vi "dl950_wave_20240509.vi"() -> ()   [LabVIEW 2019]
uses:
  950b817e-b14a-4b5d-8110-72b26e05e848.vi
  <instrlib>/Yokogawa DL950 Series/Public/Configure/Configure Module (4-CH Voltage).vi
  <instrlib>/Yokogawa DL950 Series/Public/Data/Read Waveform (Multiple).vi
  <instrlib>/Yokogawa DL950 Series/Yokogawa DL950 Series.lvlib
panel:
  out "Discharge":bool
  out "Power Relay":bool=TRUE
  out "Compute":bool
  out "DL950 Trigger":bool
  out "Power":bool=TRUE
  out "Ch 4":bool
  out "Ch 3":bool=TRUE
  out "Ch 2":bool
  out "Ch 1":bool
  in  "Channel Enale(1: CH1)":u16[](array[ring])=[1, 1] items=["", "CH1", "CH2", "CH3", "CH4", "CH5", "CH6", "CH7", "CH8", "CH9", "CH10", "CH11", "CH12", "CH13", "CH14", "CH15", "CH16", "RMATH1", "RMATH2", "RMATH3", "RMATH4", "RMATH5", "RMATH6", "RMATH7", "RMATH8", "RMATH9", "RMATH10", "RMATH11", "RMATH12", "RMATH13", "RMATH14", "RMATH15", "RMATH16"]
  in  "channel":i32[](array[ring])=[1, 2] items=["", "CH1_1", "CH1_2", "CH2_1", "CH2_2", "CH3_1", "CH3_2", "CH4_1", "CH4_2", "CH5_1", "CH5_2", "CH6_1", "CH6_2", "CH7_1", "CH7_2", "CH8_1", "CH8_2", "CH9_1", "CH9_2", "CH10_1", "CH10_2", "CH11_1", "CH11_2", "CH12_1", "CH12_2", "CH13_1", "CH13_2", "CH14_1", "CH14_2", "CH15_1", "CH15_2", "CH16_1", "CH16_2"]
  in  "trig source":i32[](array[ring])=[1, 1] items=["", "CH1", "CH2", "CH3", "CH4", "CH5", "CH6", "CH7", "CH8", "CH9", "CH10", "CH11", "CH12", "CH13", "CH14", "CH15", "CH16", "RMATH1", "RMATH2", "RMATH3", "RMATH4", "RMATH5", "RMATH6", "RMATH7", "RMATH8", "RMATH9", "RMATH10", "RMATH11", "RMATH12", "RMATH13", "RMATH14", "RMATH15", "RMATH16"]
  in  "sub channel":u16[](array[ring])=[1, 2] items=["None", "SCH1", "SCH2", "SCH3", "SCH4", "SCH5", "SCH6", "SCH7", "SCH8", "SCH9", "SCH10", "SCH11", "SCH12", "SCH13", "SCH14", "SCH15", "SCH16", "SCH17", "SCH18", "SCH19", "SCH20", "SCH21", "SCH22", "SCH23", "SCH24", "SCH25", "SCH26", "SCH27", "SCH28", "SCH29", "SCH30", "SCH31", "SCH32", "SCH33", "SCH34", "SCH35", "SCH36", "SCH37", "SCH38", "SCH39", "SCH40", "SCH41", "SCH42", "SCH43", "SCH44", "SCH45", "SCH46", "SCH47", "SCH48", "SCH49", "SCH50", "SCH51", "SCH52", "SCH53", "SCH54", "SCH55", "SCH56", "SCH57", "SCH58", "SCH59", "SCH60", "SCH61", "SCH62", "SCH63", "SCH64"]
  in  "Vertical Division (20: 50V)":i32(ring)=11 items=["0.1m", "0.2m", "0.5m", "1m", "2m", "5m", "10m", "20m", "50m", "100m", "200m", "500m", "1", "2", "4", "5", "8", "10", "20", "40", "50", "80", "100", "200", "400", "500", "800", "1k", "2k", "4k", "5k", "8k", "10k", "20k", "25k", "50k", "100k", "250k", "500k", "1000k"]
  in  "Hysteresis (1: Middle)":i32(ring)=1 items=["Low", "Middle", "High"]
  in  "Trigger Level (0)":dbl=0.4 format="%.3p"
  in  "Trigger Slope (0: Rising)":i32(ring) items=["Rising", "Falling", "Both"]
  in  "Trigger Mode (1: Auto)":i32(ring)=2 items=["Normal", "Auto", "Auto Level", "Single", "Single(N)", "On Start", "No Set"]
  in  "Time Division (12: 1ms)":i32(ring)=18 items=["100ns", "200ns", "500ns", "1us", "2us", "5us", "10us", "20us", "50us", "100us", "200us", "500us", "1ms", "2ms", "5ms", "10ms", "20ms", "50ms", "100ms", "200ms", "500ms", "1s", "2s", "3s", "4s", "5s", "6s", "10s", "20s", "30s", "1min", "2min", "3min", "4min", "5min", "6min", "10min", "12min", "30min", "1hour", "2hour", "3hour", "4hour", "5hour", "6hour", "8hour", "10hour", "12hour", "1day", "2day", "3day", "4day", "5day"]
  in  "Acquisition Mode (0: Normal)":i32(ring) items=["Normal", "Average", "Envelope"]
  in  "Record Length (0: 10k)":i32(ring) items=["10k", "25k", "50k", "100k", "250k", "500k", "1M", "2.5M", "5M", "10M", "25M", "50M", "100M", "250M", "500M", "1G", "2G", "4G", "5G", "10G", "20G", "50G"]
  in  "Sub Channel (0: None) 2":u16[](array[ring])=[1, 2] caption="Sub Channel (0: None)" items=["None", "SCH1", "SCH2", "SCH3", "SCH4", "SCH5", "SCH6", "SCH7", "SCH8", "SCH9", "SCH10", "SCH11", "SCH12", "SCH13", "SCH14", "SCH15", "SCH16", "SCH17", "SCH18", "SCH19", "SCH20", "SCH21", "SCH22", "SCH23", "SCH24", "SCH25", "SCH26", "SCH27", "SCH28", "SCH29", "SCH30", "SCH31", "SCH32", "SCH33", "SCH34", "SCH35", "SCH36", "SCH37", "SCH38", "SCH39", "SCH40", "SCH41", "SCH42", "SCH43", "SCH44", "SCH45", "SCH46", "SCH47", "SCH48", "SCH49", "SCH50", "SCH51", "SCH52", "SCH53", "SCH54", "SCH55", "SCH56", "SCH57", "SCH58", "SCH59", "SCH60", "SCH61", "SCH62", "SCH63", "SCH64"]
  in  "Source (1: CH1) 2":u16[](array[ring])=[1, 1] caption="Source (1: CH1)" items=["None", "CH1", "CH2", "CH3", "CH4", "CH5", "CH6", "CH7", "CH8", "CH9", "CH10", "CH11", "CH12", "CH13", "CH14", "CH15", "CH16", "MATH1", "MATH2", "MATH3", "MATH4", "MATH5", "MATH6", "MATH7", "MATH8", "EVENT"]
  in  "Probe Attenuation (3: 10:1)":i32(ring)=3 caption="Probe (10: 1)" items=["1:1", "2:1", "5:1", "10:1", "20:1", "50:1", "100:1", "200:1", "500:1", "1000:1", "2000:1", "5000:1", "10k:1", "20k:1", "50k:1", "0.1A:1V", "0.2A:1V", "0.5A:1V", "1A:1V", "2A:1V", "5A:1V", "10A:1V", "20A:1V", "50A:1V", "100A:1V", "200A:1V", "250A:1V", "400A:1V", "500A:1V", "1kA:1V", "2kA:1V", "5kA:1V", "10kA:1V", "20kA:1V", "50kA:1V", "NoSet"]
  in  "Vertical Coupling (1: DC)":i32(ring)=1 items=["AC", "DC", "Ground", "AC-RMS", "DC-RMS"]
  out "x-y":u32=4302
  in  "Enable Calibration (F: No)":bool
  in  "Enable Auto Setup (T: Yes)":bool
  in  "VISA resource name":refnum<visa-resource-name>="TCPIP0::192.168.0.100::inst0::INSTR"
  out "Waveform Graph":waveform(dbl)[](graph)=[{"t0"=timestamp(0 s since 1904-01-01), "dt"=0.0001, "Y"=array[10001 elements]}, {"t0"=timestamp(0 s since 1904-01-01), "dt"=0.0001, "Y"=array[10001 elements]}]
  in  "stop":bool
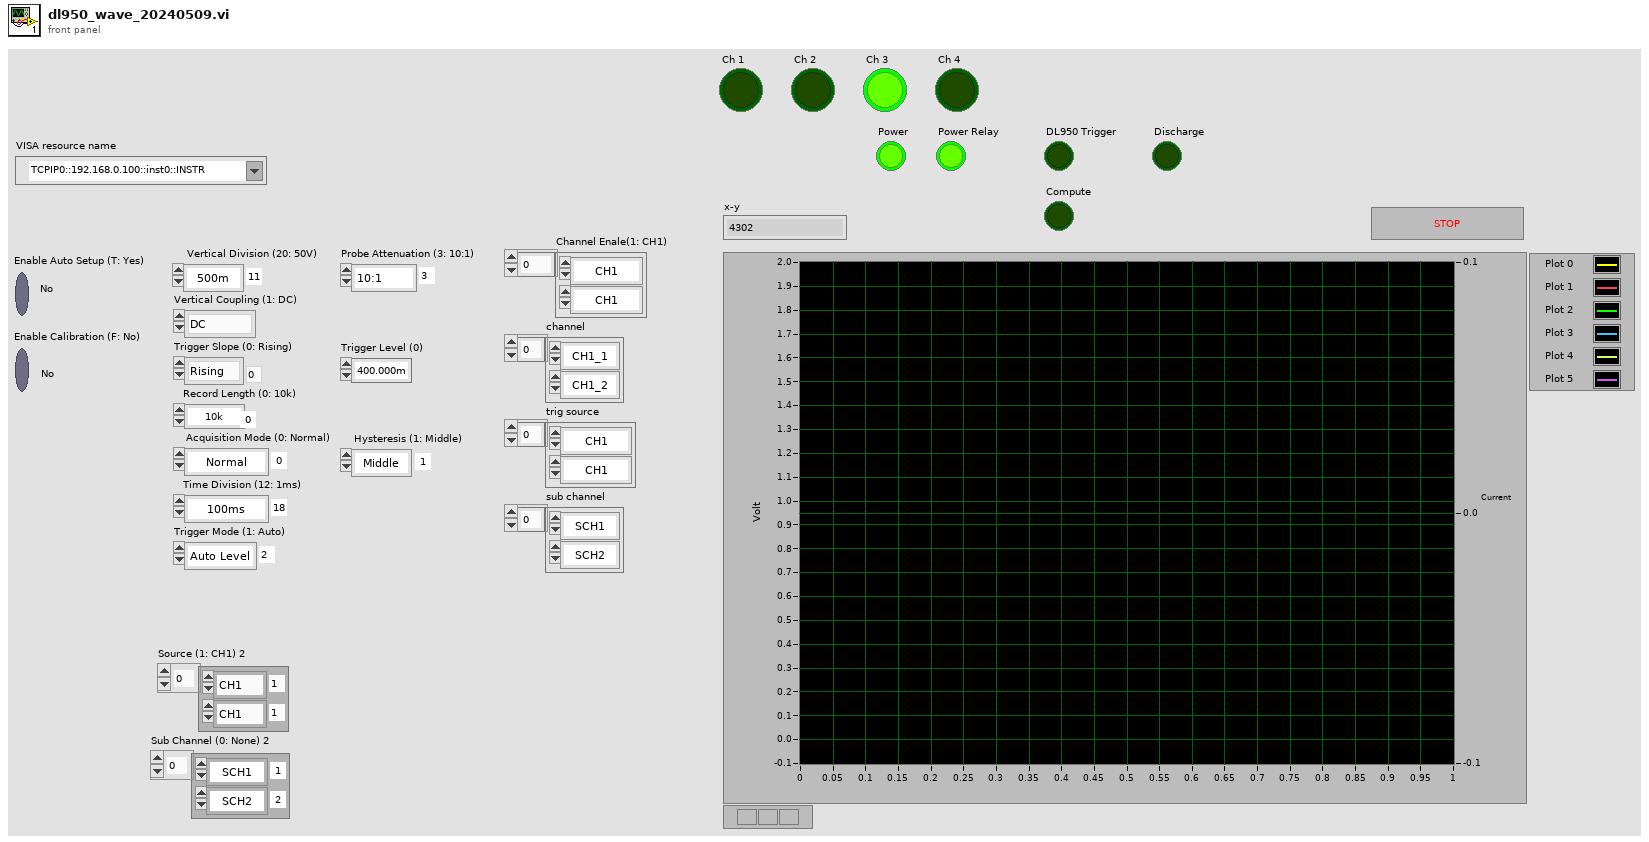
[diagram p1: front panel]
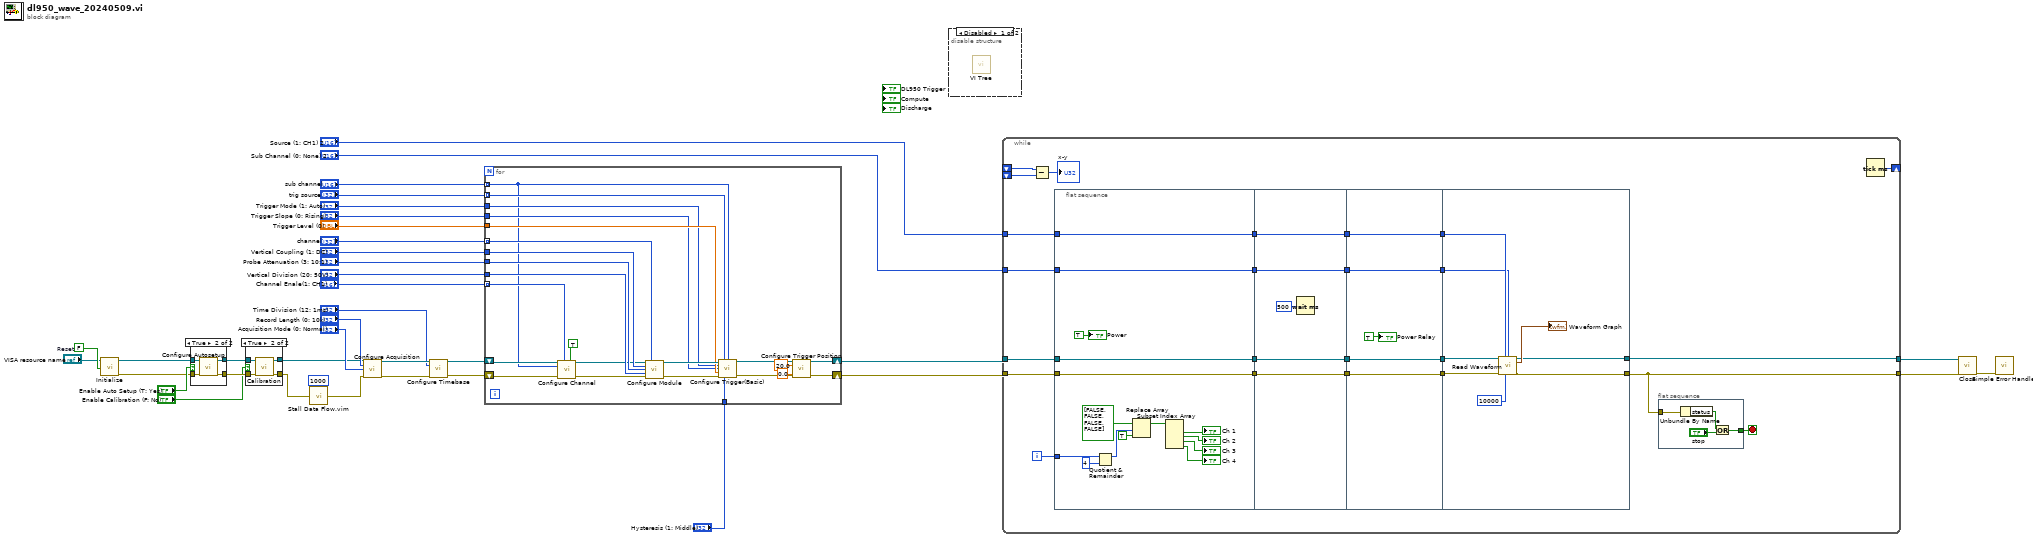
[diagram p0: block diagram]
diagram:
  w37 = FALSE  # Reset
  n1 = call <instrlib>:"Initialize.vi"("Reset (True)"=w37, "VISA resource name"="VISA resource name") -> ("error out"=w4:errorcluster, "VISA resource name out"=w5:refnum<visa-resource-name>)  [unwired: 8 in]
  n2 = case shown="True" "Enable Auto Setup (T: Yes)" {
    tunnel: w5 -> [w39 w43]
    tunnel: [w39 w42] -> w33
    tunnel: w4 -> [w38 w41]
    tunnel: [w38 w40] -> w32
    frame False {
    }
    frame True {
      n3 = call <instrlib>:"Configure Autosetup.vi"("VISA resource name"=w43, "error in (no error)"=w41) -> ("VISA resource name out"=w42:refnum<visa-resource-name>, "error out"=w40:errorcluster)  [unwired: 12 in]
    }
  }
  n4 = case shown="True" "Enable Calibration (F: No)" {
    tunnel: w33 -> [w45 w49]
    tunnel: [w45 w48] -> w3
    tunnel: w32 -> [w44 w47]
    tunnel: [w44 w46] -> w2
    frame False {
    }
    frame True {
      n5 = call <instrlib>:"Calibration.vi"("error in (no error)"=w47, "VISA resource name"=w49) -> ("error out"=w46:errorcluster, "VISA resource name out"=w48:refnum<visa-resource-name>)  [unwired: 8 in]
    }
  }
  n6 = call "Stall Data Flow.vim"("value in"=w2, "milliseconds to wait"=u32 1000) -> ("value out"=w1:errorcluster)  [unwired: 1 out]
  n7 = call <instrlib>:"Configure Acquisition.vi"("VISA resource name"=w3, "Record Length (0: 10k)"="Record Length (0: 10k)", "Acquisition Mode (0: Normal)"="Acquisition Mode (0: Normal)", "error in (no error)"=w1) -> ("VISA resource name out"=w24:refnum<visa-resource-name>, "error out"=w23:errorcluster)  [unwired: 10 in]
  n8 = call <instrlib>:"Configure Timebase.vi"("VISA resource name"=w24, "Time Division (12: 1ms)"="Time Division (12: 1ms)", "error in (no error)"=w23) -> ("VISA resource name out"=w22:refnum<visa-resource-name>, "error out"=w21:errorcluster)  [unwired: 11 in]
  n9 = for {
    tunnel: "channel" -> [w60] mode=indexing
    tunnel: "trig source" -> [w73] mode=indexing
    tunnel: "sub channel" -> [w56] mode=indexing
    tunnel: "Hysteresis (1: Middle)" -> [w72]
    shift-right: [w54] -> w7
    shift-left: w22 -> [w63]
    shift-right: [w52] -> w6
    shift-left: w21 -> [w61]
    tunnel: "Trigger Level (0)" -> [w69]
    tunnel: "Trigger Slope (0: Rising)" -> [w68]
    tunnel: "Trigger Mode (1: Auto)" -> [w67]
    tunnel: "Vertical Division (20: 50V)" -> [w66]
    tunnel: "Probe Attenuation (3: 10:1)" -> [w65]
    tunnel: "Vertical Coupling (1: DC)" -> [w64]
    tunnel: "Channel Enale(1: CH1)" -> [w58] mode=indexing
    n10 = call <instrlib>:"Configure Channel.vi"("VISA resource name"=w63, "Channel (1: CH1)"=w58, "Enable Channel (True)"=TRUE, "sub Channel (1: CH1)"=w56, "error in (no error)"=w61) -> ("VISA resource name out"=w62:refnum<visa-resource-name>, "error out"=w59:errorcluster)  [unwired: 9 in]
    n11 = call-poly <instrlib>:"Configure Module.vi"("VISA resource name"=w62, "Channel (1: CH1_1)"=w60, "Vertical Coupling (1: DC)"=w64, "Probe Attenuation (3: 10:1)"=w65, "Vertical Division (20: 50V)"=w66, "error in (no error)"=w59) -> ("VISA resource name out"=w71:refnum<visa-resource-name>, "error out"=w70:errorcluster)  [unwired: 8 in]
    n12 = call <instrlib>:"Configure Trigger(Basic).vi"("VISA resource name"=w71, "Trigger Source (1: CH1)"=w73, "Sub Channel (0: None)"=w56, "Trigger Mode (1: Auto)"=w67, "Trigger Slope (0: Rising)"=w68, "Trigger Level (0)"=w69, "error in (no error)"=w70, "Hysteresis (1: Middle)"=w72) -> ("VISA resource name out"=w55:refnum<visa-resource-name>, "error out"=w53:errorcluster)  [unwired: 6 in]
    n13 = call <instrlib>:"Configure Trigger Position.vi"("VISA resource name"=w55, "Trigger Position (50%)"=20.0, "Trigger Delay (0.0000000s)"=0.0, "error in (no error)"=w53) -> ("VISA resource name out"=w54:refnum<visa-resource-name>, "error out"=w52:errorcluster)  [unwired: 10 in]
  }
  n14 = disable-structure shown="Disabled" {
    frame Disabled {
      n15 = call <instrlib>:"VI Tree.vi"() -> ()  [unwired: 12 in]
    }
    frame Enabled {
    }
  }
  n16 = while "Whileループ" {
    shift-right: [w96] -> _
    shift-left: _ -> [w95]
    shift-left: _ -> [w94]
    tunnel: w7 -> [w92]
    tunnel: w6 -> [w91]
    tunnel: "Source (1: CH1) 2" -> [w90]
    tunnel: "Sub Channel (0: None) 2" -> [w89]
    tunnel: [w88] -> w9
    tunnel: [w87] -> w8
    i -> [w86]
    stop <- w97 stop-if-true
    n17 = Subtract(x=w95, y=w94) -> (x-y=→"x-y":u32)
    n18 = flat-sequence {
      tunnel: w92 -> [w111]
      tunnel: w91 -> [w110]
      tunnel: w90 -> [w109]
      tunnel: w89 -> [w108]
      tunnel: [w111] -> w85
      tunnel: [w110] -> w84
      tunnel: [w109] -> w83
      tunnel: [w108] -> w82
      tunnel: w86 -> [w98]
      tunnel: w85 -> [w117]
      tunnel: [w117] -> w81
      tunnel: w84 -> [w116]
      tunnel: [w116] -> w79
      tunnel: w83 -> [w115]
      tunnel: [w115] -> w77
      tunnel: w82 -> [w114]
      tunnel: [w114] -> w75
      tunnel: w81 -> [w122]
      tunnel: [w122] -> w80
      tunnel: w79 -> [w121]
      tunnel: [w121] -> w78
      tunnel: w77 -> [w120]
      tunnel: [w120] -> w76
      tunnel: w75 -> [w119]
      tunnel: [w119] -> w74
      tunnel: w80 -> [w127]
      tunnel: w78 -> [w126]
      tunnel: w76 -> [w129]
      tunnel: w74 -> [w128]
      tunnel: [w124] -> w88
      tunnel: [w123] -> w87
      frame #0 {
        n19 = Quotient & Remainder(x=w98, y=4) -> (x-y*floor(x/y)=w107:i32)  [unwired: 1 out]
        n20 = Replace Array Subset(array=bool[] [FALSE, FALSE, FALSE, FALSE], new element=TRUE ("new element/subarray"), index=w107) -> (w106:bool[])
        n21 = Index Array(array=w106) -> (element #1=→"Ch 1":bool, element #2=→"Ch 2":bool, element #3=→"Ch 3":bool, element #4=→"Ch 4":bool)  [unwired: 4 in]
        "Power" <- TRUE ("Power")
      }
      frame #1 {
        n22 = Wait (ms)(milliseconds to wait=u32 500) -> ()  [unwired: 1 out]
      }
      frame #2 {
        "Power Relay" <- TRUE ("Power Relay")
      }
      frame #3 {
        n23 = call-poly <instrlib>:"Read Waveform.vi"("VISA resource name"=w127, "Source (1: CH1)"=w129, "Sub Channel (0: None)"=w128, "error in (no error)"=w126, "Timeout (10000 ms)"=u32 10000) -> ("VISA resource name out"=w124:refnum<visa-resource-name>, "Waveform Data"=→"Waveform Graph":waveform(dbl)[], "error out"=w123:errorcluster)  [unwired: 8 in]
      }
    }
    n24 = flat-sequence {
      tunnel: [w133] -> w97
      tunnel: w87 -> [w131]
      frame #0 {
        n25 = Unbundle By Name ("名前でバンドル解除")(w131) -> ("status"=w132:bool)
        n26 = Or(x=w132, y="stop") -> (x .or. y?=w133:bool)
      }
    }
    n27 = Tick Count (ms)() -> (millisecond timer value=w96:u32)
  }
  n28 = call <instrlib>:"Close.vi"("error in (no error)"=w8, "VISA resource name"=w9) -> ("error out"=w36:errorcluster)  [unwired: 9 in]
  n29 = call <vilib>:"Simple Error Handler.vi"("error in (no error)"=w36) -> ()  [unwired: 4 in, 5 out]
